vi "Cleanup.vi"(8 "error in (no error)":errorcluster, 11 "LightsPanel in":refnum<class "LightsPanel.lvclass">) -> (0 "error out":errorcluster)   [LabVIEW 2022 SP3, in "TouchControl.lvlib" / "LightsPanel.lvclass"]
uses:
  LightsPanel.lvclass
  LightsPanel.lvclass/LightsPanel.ctl
  <vilib>/IlluminatedG/IG OOPanel/OOPanel/Panel/Panel.lvclass
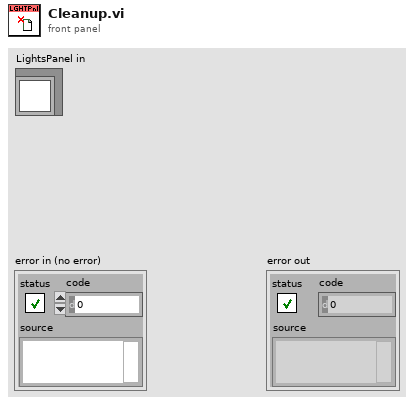
[diagram p1: front panel]
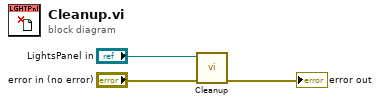
[diagram p0: block diagram]
diagram:
  n1 = call-parent "Cleanup.vi"("error in (no error)"="error in (no error)", "Panel in"="LightsPanel in") -> ("error out"=→"error out":errorcluster)  [unwired: 9 in]
